vi "TM Init and Last.vi"(11 "List":string[](array[string])) -> (2 "Last":string, 3 "Init List":string[](array[string]))   [LabVIEW 2021, in "Tree Map.lvlib"]
doc: "Init List - Return all but the last element of the list. \nLast - Returns the last element of the list.\nAdapts to wired data types."
uses:
  <vilib>/National Instruments/Tree Map/Tree Map.lvlib
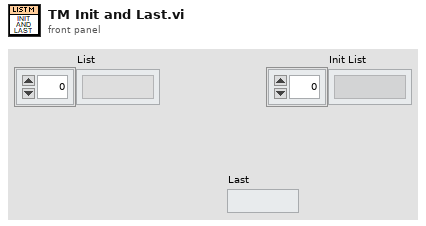
[diagram p1: front panel]
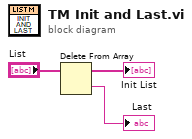
[diagram p0: block diagram]
diagram:
  n1 = Delete From Array(array="List") -> (deleted portion=→"Last":string, array with subset deleted=→"Init List":string[])  [unwired: 2 in]
